vi "LMData_measure.vi"(8 "error in (no error)":errorcluster, 9 "MeasurementInterval(>0)":i64, 10 "MeasurementIndex":i64, 11 "LMData in":refnum<class "LMData.lvclass">) -> (0 "error out":errorcluster, 1 "LastDataArray":dbl[][](array[numeric]), 2 "LastMeasurement":dbl[](array[numeric]), 3 "LMData out":refnum<class "LMData.lvclass">, 5 "LastTimeArray":timestamp[](array[timestamp]))   [LabVIEW 2017, in "LMData.lvclass"]
uses:
  LMData.lvclass
  LMData.lvclass/LMData.ctl
  <instrlib>/Agilent 34401/Public/Data/Read (Single Point).vi
  <vilib>/express/express arith-compare/Formula/XNode/ExpressFormulaBlockNode.xnode
  <instrlib>/Agilent 34401/Agilent 34401.lvlib
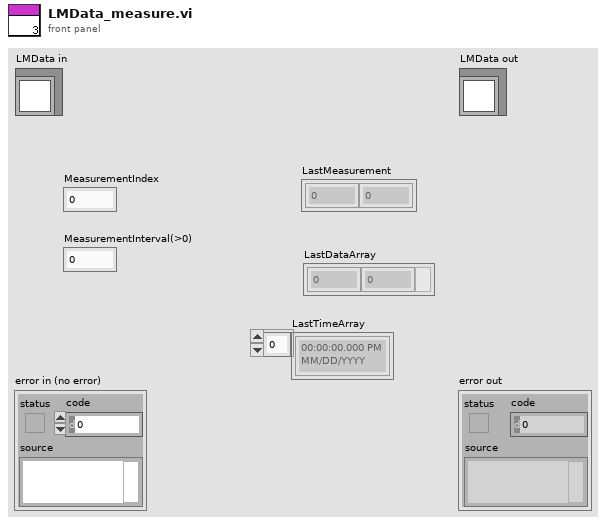
[diagram p1: front panel]
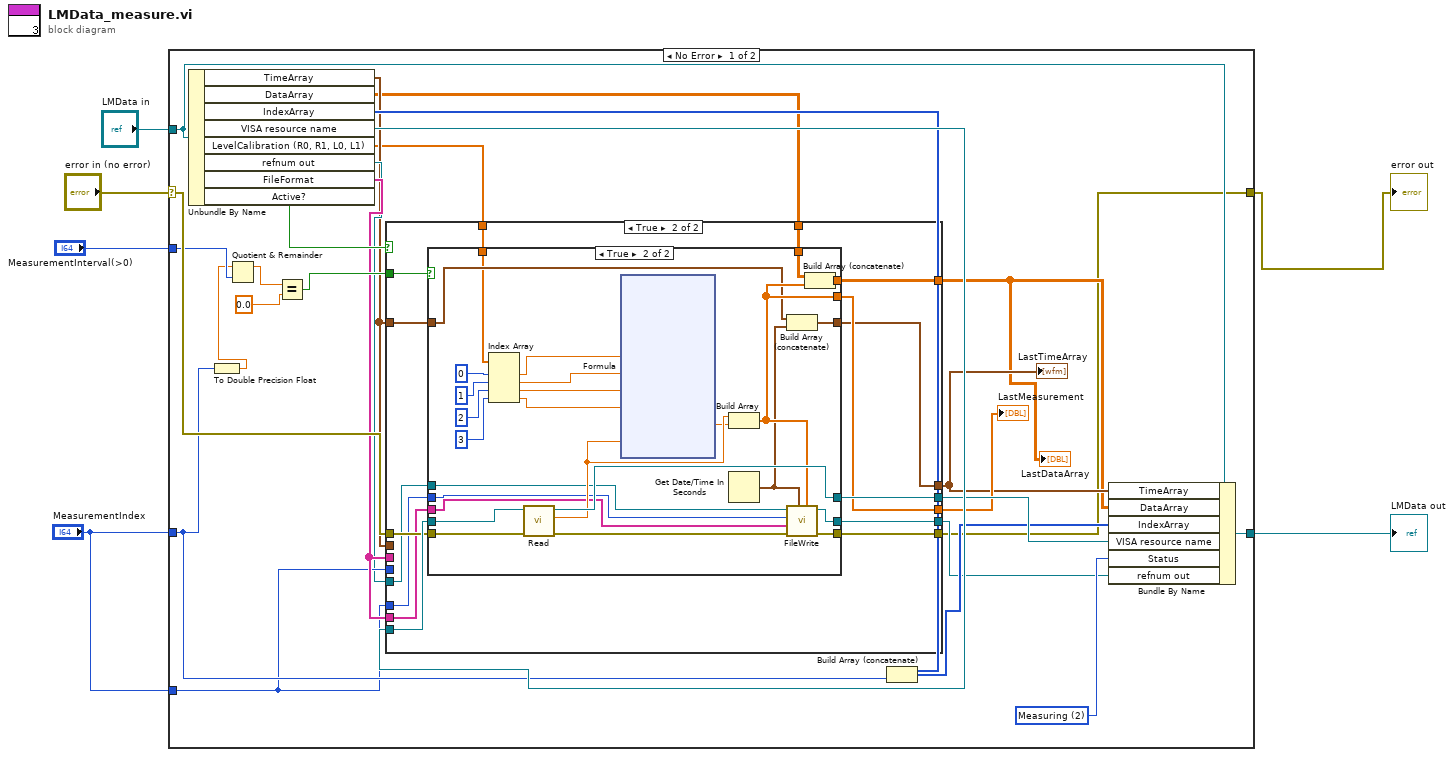
[diagram p0: block diagram]
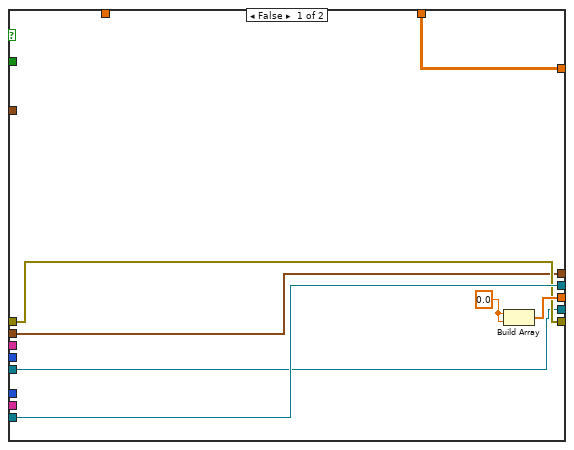
[diagram p2: hidden frame]
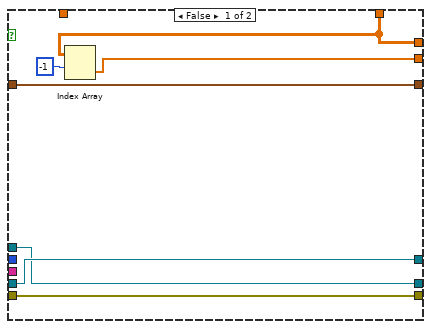
[diagram p3: hidden frame]
diagram:
  n1 = case shown="No Error" "error in (no error)" {
    selector: "error in (no error)" -> [w31 w105]
    tunnel: [w7 w105] -> w1
    tunnel: [w29 w104] -> w4
    tunnel: "LMData in" -> [w30 w104]
    tunnel: "MeasurementIndex" -> [w21 _]
    tunnel: "MeasurementInterval(>0)" -> [w23 _]
    tunnel: "MeasurementIndex" -> [w15 _]
    frame No Error {
      w25 = u16 2 items=["Initialized", "Waiting", "Measuring", "Terminated"] ("Status")
      n2 = Unbundle By Name(w30) -> ("TimeArray"=w12:timestamp[], "DataArray"=w10:dbl[][], "IndexArray"=w27:i64[], "VISA resource name"=w32:refnum<visa-resource-name>, "LevelCalibration (R0, R1, L0, L1)"=w8:dbl[], "refnum out"=w14:refnum<file>, "FileFormat"=w16:string[], "Active?"=w24:bool)
      n3 = To Double Precision Float(number=w21) -> (double precision float=w20:dbl)
      n4 = Quotient & Remainder(x=w20, y=w23) -> (x-y*floor(x/y)=w19:dbl)  [unwired: 1 out]
      n5 = Equal?(x=w19, y=0.0) -> (x = y?=w18:bool)
      n6 = case shown="True" w24 {
        tunnel: w32 -> [w38 w54]
        tunnel: w31 -> [w36 w53]
        tunnel: [w38 w52] -> w28
        tunnel: w18 -> [_ w51]
        tunnel: w12 -> [w35 _]
        tunnel: w16 -> [_ _]
        tunnel: w15 -> [_ _]
        tunnel: w14 -> [w34 w43]
        tunnel: [w37 w50] -> w17
        tunnel: w16 -> [_ w49]
        tunnel: w15 -> [_ w48]
        tunnel: [w36 w46] -> w7
        tunnel: [w34 w47] -> w13
        tunnel: w12 -> [_ w45]
        tunnel: [w35 w44] -> w11
        tunnel: w10 -> [w33 w42]
        tunnel: [w33 w41] -> w9
        tunnel: w8 -> [_ w40]
        frame False {
          w39 = 0.0 ("element")
          n7 = Build Array(w39, w39) -> (w37:dbl[])
        }
        frame True {
          n8 = case shown="True" w51 {
            tunnel: w54 -> [w59 w87]
            tunnel: w53 -> [w61 w86]
            tunnel: [w59 w85] -> w52
            tunnel: [w55 w78] -> w50
            tunnel: [w61 w69] -> w46
            tunnel: w49 -> [_ w76]
            tunnel: w48 -> [_ w75]
            tunnel: w43 -> [w58 w74]
            tunnel: [w58 w73] -> w47
            tunnel: w45 -> [w57 w72]
            tunnel: [w57 w70] -> w44
            tunnel: w42 -> [w56 w68]
            tunnel: [w56 w67] -> w41
            tunnel: w40 -> [_ w66]
            frame False {
              n9 = Index Array(array=w56, index (row)=-1) -> (element=w55:dbl[])  [unwired: 1 in]
            }
            frame True {
              n10 = Index Array(array=w66, index #1=0 ("index"), index #2=1 ("index"), index #3=2 ("index"), index #4=3 ("index")) -> (element #1=w65:dbl, element #2=w64:dbl, element #3=w63:dbl, element #4=w62:dbl)
              n11 = call-poly <instrlib>:"Read.vi"("error in (no error)"=w86, "VISA resource name"=w87) -> ("error out"=w77:errorcluster, "Measurement"=w84:dbl, "VISA resource name out"=w85:refnum<visa-resource-name>)  [unwired: 7 in]
              n12 = xnode "Formula"("X0"=w65, "X1"=w64, "Y0"=w63, "Y1"=w62, "X"=w84) -> ("Result"=w83:dbl)  [unwired: 1 in, 1 out]
              n13 = Build Array(w84, w83) -> (w78:dbl[])
              n14 = Get Date/Time In Seconds() -> (seconds since 1Jan1904=w71:timestamp)
              n15 = Build Array (concatenate)(w72, w71) -> (w70:timestamp[])
              n16 = call "FileWrite.vi"("DataArray"=w78, "Time Stamp"=w71, "Error In"=w77, "FileFormat"=w76, "Index"=w75, "refnum in"=w74) -> ("Error Out"=w69:errorcluster, "Byte Stream File Refnum"=w73:refnum<file>)  [unwired: 4 in]
              n17 = Build Array (concatenate)(w68, w78) -> (w67:dbl[][])
            }
          }
        }
      }
      "LastDataArray" <- w9
      "LastTimeArray" <- w11
      "LastMeasurement" <- w17
      n18 = Build Array (concatenate)(w27, w21) -> (w26:i64[])
      n19 = Bundle By Name(cluster=w30, "TimeArray"=w11, "DataArray"=w9, "IndexArray"=w26, "VISA resource name"=w28, "Status"=w25, "refnum out"=w13) -> (w29:refnum<class "LMData.lvclass">)
    }
    frame Error {
    }
  }
  "error out" <- w1
  "LMData out" <- w4
